vi "NISE.local.Get NVMEM Bytes.vi"(0 "SLSC Local In":refnum<class "SLSC Interface.lvclass">, 5 "NVMEM area":refnum<k21>="$DefaultNVMEMAreas", 7 "data address":u32 format="%.0x", 9 "data size":u32, 11 "error in (no error)":errorcluster) -> (4 "SLSC Local Out":refnum<class "SLSC Interface.lvclass">, 6 "NVMEM area out":refnum<k21>, 8 "next data address":u32 format="%.0x", 10 "data out":u8[](array[numeric]) format="%.0x", 15 "error out":errorcluster)   [LabVIEW 2016, in "SLSC Interface.lvclass"]
uses:
  SLSC Interface Class/SLSC Interface.lvclass
  SLSC Interface Class/NISE.Read session.vi
  SLSC Interface Class/NISE.Write session.vi
  <vilib>/SLSC/SLSC.lvlib
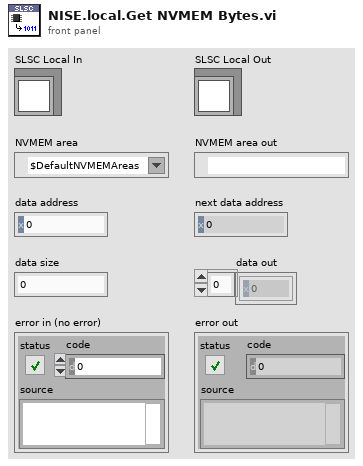
[diagram p1: front panel]
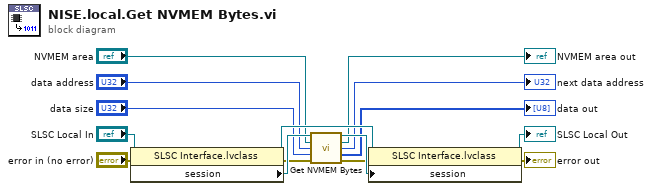
[diagram p0: block diagram]
diagram:
  n1 = property class="SLSC Interface.lvclass"(reference="SLSC Local In", error in="error in (no error)") -> (reference out=w14:refnum<class "SLSC Interface.lvclass">, error out=w3:errorcluster, "session"=w12:refnum<k21>)
  n2 = call <vilib>:"Get NVMEM Bytes.vi"("session in"=w12, "NVMEM area"="NVMEM area", "data address"="data address", "data size"="data size", "error in (no error)"=w3) -> ("session out"=w11:refnum<k21>, "NVMEM area out"=→"NVMEM area out":refnum<k21>, "next data address"=→"next data address":u32, "data out"=→"data out":u8[], "error out"=w2:errorcluster)  [unwired: 6 in]
  n3 = property class="SLSC Interface.lvclass"(reference=w14, error in=w2, "session"=w11) -> (reference out=→"SLSC Local Out":refnum<class "SLSC Interface.lvclass">, error out=→"error out":errorcluster)
